vi "Get Time Stamp.vi"(11 "CANopen Message in":refnum<class "CANopen Message.lvclass">) -> (2 "Time Stamp":refnum<class "Time Stamp.lvclass">, 3 "CANopen Message out":refnum<class "CANopen Message.lvclass">)   [LabVIEW 2024, in "CANopen Master.lvlib" / "CANopen Message.lvclass"]
uses:
  CANopen Message.lvclass
  CANopen Message.lvclass/CANopen Message.ctl
  HAL/HAL/Time Stamp/Time Stamp.lvclass
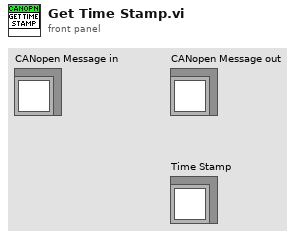
[diagram p1: front panel]
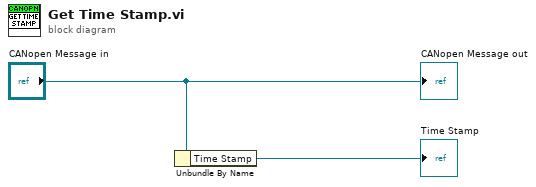
[diagram p0: block diagram]
diagram:
  n1 = Unbundle By Name("CANopen Message in") -> ("Time Stamp"=→"Time Stamp":refnum<class "Time Stamp.lvclass">)
  "CANopen Message out" <- "CANopen Message in"
